vi "Barcode-Indentify-Read_Api.vi"(8 "Error In":errorcluster, 11 "Progressing Data":T3) -> (0 "Error Out":errorcluster, 2 "Barcodes":T4(array[cluster]) {"Confidence Level" format="%.2f"; "Barcode Type" items=["Reserved", "Codabar", "Code 39", "Code 93", "Code 128", "EAN 8", "EAN 13", "Interleaved 2 of 5", "MSI", "UPCA", "Pharmacode", "RSS Limited"]; "Bounding Box"."y" format="%.2f"; "Bounding Box"."x" format="%.2f"}, 3 "Progressing Data":T3, 5 "Image":T1(plugin-control))   [LabVIEW 2019]
uses:
  <vilib>/vision/Image Controls.llb/IMAQ Image.ctl
  <vilib>/userDefined/High Color/IMAQdx.ctl
  <vilib>/vision/Instrument.llb/Barcode Search Options.ctl
  <vilib>/vision/driver/NI_Vision_Acquisition_Software.lvlib
  <vilib>/vision/NI_Vision_Development_Module.lvlib
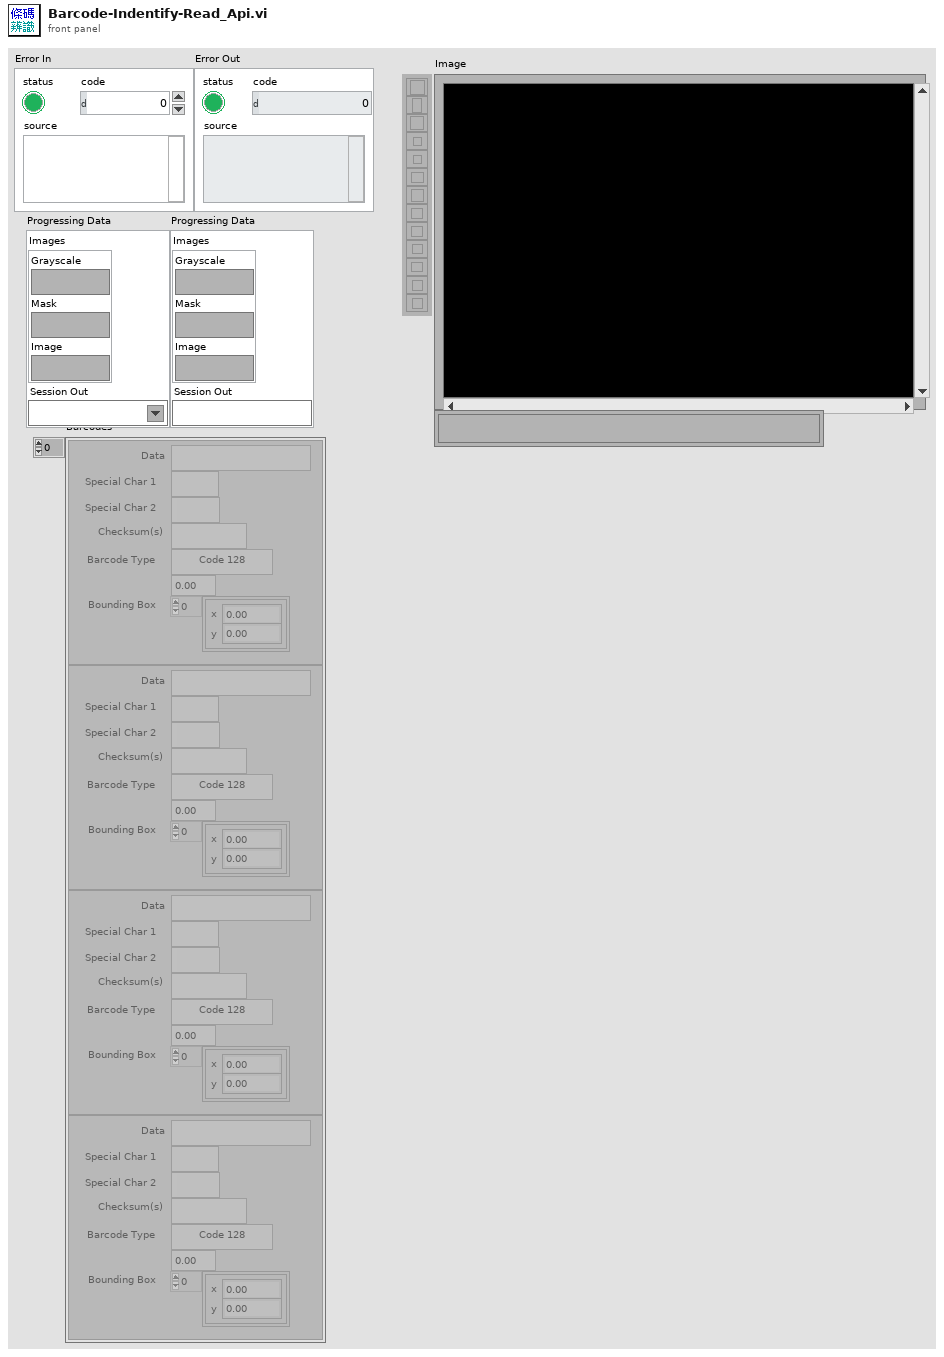
[diagram p1: front panel]
types:
  T1 = typedef "IMAQ Image.ctl" = refnum<image>
  T2 = typedef "IMAQdx.ctl" = refnum<k21>
  T3 = cluster{"Images":cluster{"Grayscale":T1, "Mask":T1, "Image":T1}, "Session Out":T2}
  T4 = cluster{"Data":string, "Special Char 1":string, "Special Char 2":string, "Checksum(s)":string, "Barcode Type":u32, "Confidence Level":sgl, "Bounding Box":cluster{"x":sgl, "y":sgl}[]}[]
  T5 = typedef "Barcode Search Options.ctl" = cluster{"Min Bar Width":u32, "Min Edge Strength":u32, "Min Bars":u32, "Skip Location Search?":bool}
  T6 = typedef "IMAQ Rectangle" = cluster{"Left":i32, "Top":i32, "Right":i32, "Bottom":i32, "Rotation":dbl}
  T7 = typedef "ROI Descriptor" = cluster{"Global Rectangle":i32[], "Contours":cluster{"ID":enum32{"External", "Internal"}, "Type":u32, "Coordinates":i32[]}[]}
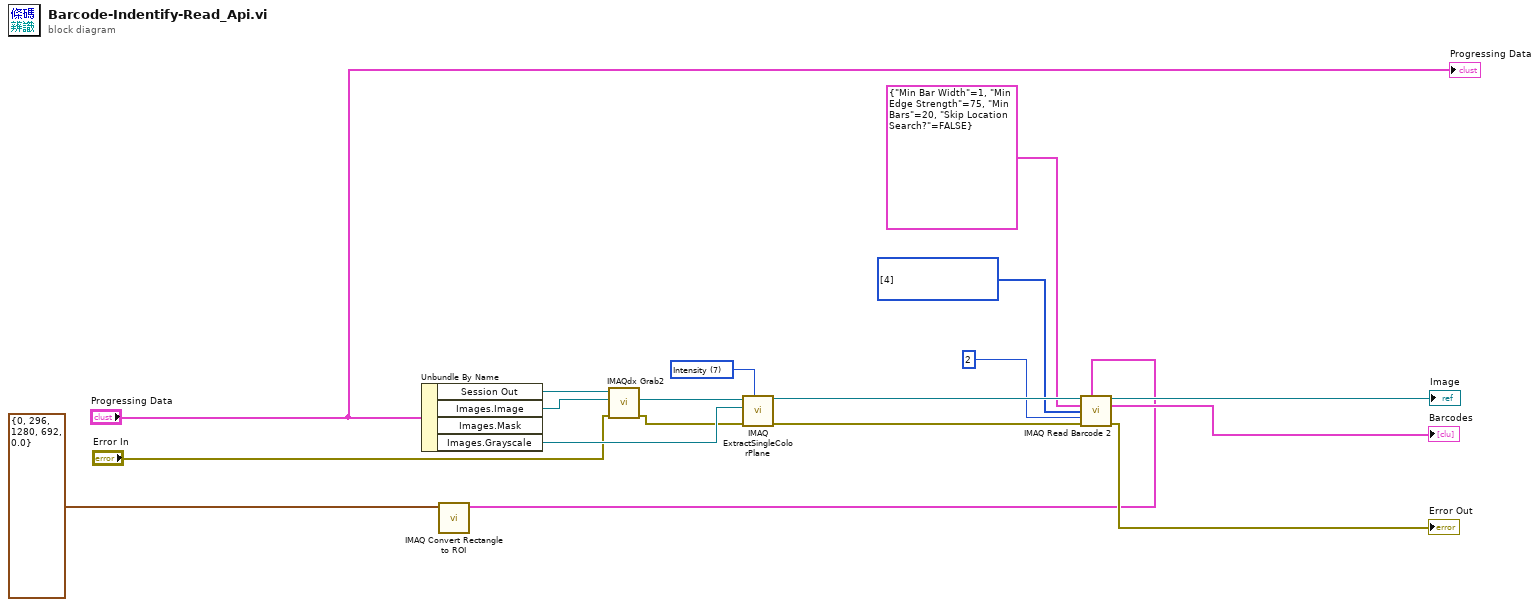
[diagram p0: block diagram]
diagram:
  w4 = 7 items=["Red", "Green", "Blue", "Hue", "Saturation", "Luminance", "Value", "Intensity"] ("Color Plane")
  w6 = u32[] [4] items=["Reserved", "Codabar", "Code 39", "Code 93", "Code 128", "EAN 8", "EAN 13", "Interleaved 2 of 5", "MSI", "UPCA", "Pharmacode", "RSS Limited"] ("Barcode Types To Search")
  n1 = Unbundle By Name("Progressing Data") -> ("Session Out"=w3:T2, "Images.Image"=w13:T1, "Images.Grayscale"=w12:T1)  [unwired: 1 out]
  n2 = call "IMAQ Convert Rectangle to ROI"("Rectangle"=T6 {"Left"=0, "Top"=296, "Right"=1280, "Bottom"=692, "Rotation"=0.0}) -> ("ROI Descriptor"=w2:T7)  [unwired: 8 in, 1 out]
  n3 = call <vilib>:"IMAQdx Grab2.vi"("error in"="Error In", "Image In"=w13, "Session In"=w3) -> ("error out"=w11:errorcluster, "Image Out"=w10:T1)  [unwired: 5 in, 2 out]
  n4 = call "IMAQ ExtractSingleColorPlane"("Color Plane"=w4, "error in (no error)"=w11, "Image Dst"=w12, "Image Src"=w10) -> ("error out"=w9:errorcluster, "Image Dst Out"=w8:T1)  [unwired: 6 in]
  n5 = call "IMAQ Read Barcode 2"("Image"=w8, "ROI Descriptor"=w2, "Barcode Search Options"=T5 {"Min Bar Width"=1, "Min Edge Strength"=75, "Min Bars"=20, "Skip Location Search?"=FALSE}, "Barcode Types To Search"=w6, "Num of Required Barcodes"=u32 2, "error in (no error)"=w9) -> ("Image (duplicate)"=→"Image":T1, "Barcodes"=→"Barcodes":T4, "error out"=→"Error Out":errorcluster)  [unwired: 5 in, 2 out]
  "Progressing Data" <- "Progressing Data"
